vi "FileExist.vi"(8 "error in (no error)":errorcluster caption="错误输入（无错误）", 11 "FilePath":string) -> (0 "error out":errorcluster caption="错误输出", 3 "exists?":bool caption="文件或文件夹存在？")   [LabVIEW 2014]
panel:
  out "路径":path
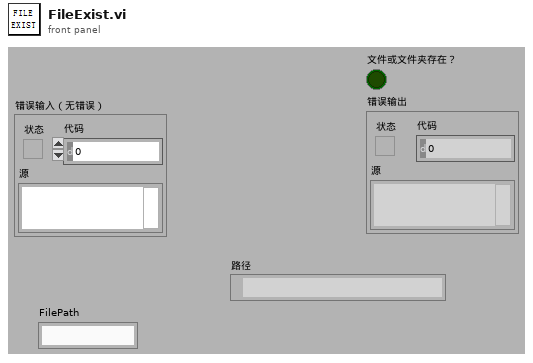
[diagram p1: front panel]
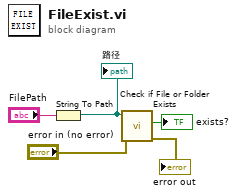
[diagram p0: block diagram]
diagram:
  n1 = String To Path(string="FilePath") -> (path=w5:path)
  "路径" <- w5
  n2 = call <vilib>:"Check if File or Folder Exists.vi"("error in (no error)"="error in (no error)", "path"=w5) -> ("error out"=→"error out":errorcluster, "file or folder exists?"=→"exists?":bool)  [unwired: 7 in, 1 out]
